vi "Configure Protection WDOG State and Delay.vi"(8 "error in":errorcluster, 9 "WDOG Delay(S)":dbl=2.0 min=2.0 max=3600.0, 10 "State":bool, 11 "VISA resource name":refnum<visa-resource-name>) -> (0 "error out":errorcluster, 3 "VISA resource name out":refnum<visa-resource-name>)   [LabVIEW 2018, in "IT-M3100.lvlib"]
doc: "This command sets the communications watchdog status and time.\n<b>State</b>\n0:Close the State\n1:Open the state\n<b>WDOG Delay(S)</b>\n2-3600"
uses:
  IT-M3100.lvlib
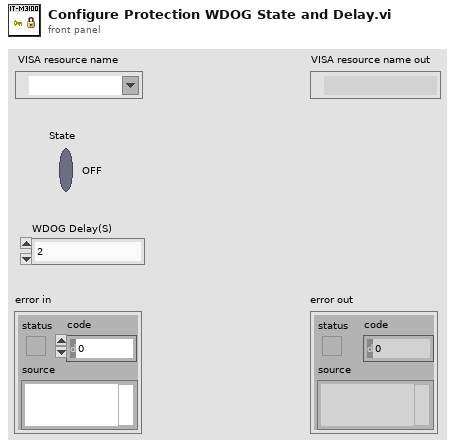
[diagram p1: front panel]
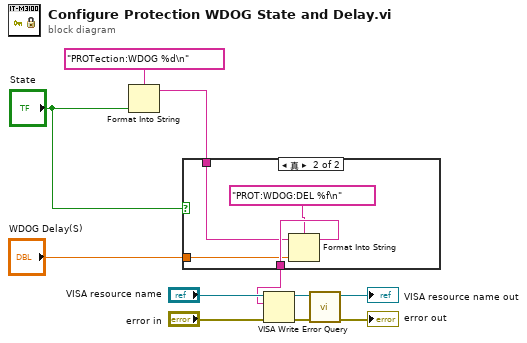
[diagram p0: block diagram]
diagram:
  n1 = Format Into String(format string="PROTection:WDOG %d\n", "State") -> (resulting string=w3:string)  [unwired: 2 in, 1 out]
  n2 = case shown="真" "State" {
    tunnel: w3 -> [w12 w14]
    tunnel: [w12 w16] -> w4
    tunnel: "WDOG Delay(S)" -> [_ w13]
    frame False {
    }
    frame True {
      n3 = Format Into String(format string="PROT:WDOG:DEL %f\n", initial string=w14, w13) -> (resulting string=w16:string)  [unwired: 1 in, 1 out]
    }
  }
  n4 = VISA Write(VISA resource name="VISA resource name", write buffer=w4, error in (no error)="error in") -> (VISA resource name out=w8:refnum<visa-resource-name>, error out=w9:errorcluster)  [unwired: 1 out]
  n5 = call "Error Query.vi"("error in"=w9, "VISA resource name"=w8) -> ("error out"=→"error out":errorcluster, "VISA resource name out"=→"VISA resource name out":refnum<visa-resource-name>)  [unwired: 6 in, 2 out]
